vi "charudatta.vi"() -> ()   [LabVIEW 2012]
uses:
  <vilib>/addons/Modulation/Digital/General/MT Generate PSK System Parameters(M).vi
  <instrlib>/niUSRP/niUSRP Write Tx Data (CDB Cluster).vi
  <vilib>/addons/Modulation/Digital/General/MT Generate Bits (Galois, PN Order).vi
  <vilib>/addons/Modulation/niDMT.lvlib
panel:
  out "error out 2":errorcluster caption="error out"
  out "Symbol Rate":dbl
  out "Number of Packets":i32
  in  "Tab Control":T1(tab)
  in  "Message Text":string="Two roads diverged in a yellow wood,\nAnd sorry I could not travel both\nAnd be one traveler, long I stood\nAnd looked down one as far as I could\nTo where it bent in the undergrowth.\n\nThen took the other, as just as fair,\nAnd having perhaps the better claim,\nBecause it was grassy and wanted wear;\nThough as for that the passing there\nHad worn them really about the same.\n\nAnd both that morning equally lay\nIn leaves no step had trodden black.\nOh, I kept the first for another day!\nYet knowing how way leads on to way,\nI doubted if I should ever come back.\n\nI shall be telling this with a sigh\nSomewhere ages and ages hence:\nTwo roads diverged in a wood, and I--\nI took the one less traveled by,\nAnd that has made all the difference.\n"
  in  "Packet Parameters":T2={"Guard Bits "=30, "Sync Bits"=20, "Message Bits"=128}
  in  "Packet Pad \n[samples]":i32=200
  in  "Blank Frame \n[samples]":i32=500
  out "Number of Packets in Message":i32=46
  in  "PN sequence order\nfor Sync Bits":i32=31 caption="PN sequence order (9)"
  in  "Packet Repeat":i32=2
  in  "Select PSK Modulation Format":T3(tab)=enum."QPSK" caption="PSK"
  in  "BPSK System Parameters":T4={"Samples per Symbol"=8, "symbol map"=[], "Differential PSK"=enum."disable", "PSK type"=0} {"PSK type" items=["normal", "shifted", "offset"]; "symbol map" format="%.3f"}
  in  "QPSK System Parameters":T4={"Samples per Symbol"=8, "symbol map"=[], "Differential PSK"=enum."disable", "PSK type"=0} {"PSK type" items=["normal", "shifted", "offset"]; "symbol map" format="%.3f"}
  in  "pi/4 DQPSK System Parameters":T4={"Samples per Symbol"=8, "symbol map"=[], "Differential PSK"=enum."enable", "PSK type"=1} {"PSK type" items=["normal", "shifted", "offset"]; "symbol map" format="%.3f"}
  in  "OQPSK System Parameters":T4={"Samples per Symbol"=8, "symbol map"=[], "Differential PSK"=enum."disable", "PSK type"=2} {"PSK type" items=["normal", "shifted", "offset"]; "symbol map" format="%.3f"}
  in  "8-PSK System Parameters":T4={"Samples per Symbol"=8, "symbol map"=[], "Differential PSK"=enum."disable", "PSK type"=0} {"PSK type" items=["normal", "shifted", "offset"]; "symbol map" format="%.3f"}
  in  "16-PSK System Parameters":T4={"Samples per Symbol"=8, "symbol map"=[], "Differential PSK"=enum."disable", "PSK type"=0} {"PSK type" items=["normal", "shifted", "offset"]; "symbol map" format="%.3f"}
  in  "M":i32=4 min=2 step=2
  in  "Custom System Parameters":T4={"Samples per Symbol"=8, "symbol map"=[], "Differential PSK"=enum."disable", "PSK type"=0} {"PSK type" items=["normal", "shifted", "offset"]; "symbol map" format="%.3f"}
  in  "Pulse Shaping Filter Parameters":T5={"Alpha"=0.5, "Filter Length"=6, "TX Filter"=enum."Root Raised Cos"} caption="Pulse Shaping Filter" {"Alpha" format="%.2f"}
  in  "Tx Parameters":T6={"Tx IQ Sampling\nRate [s/sec]"=500000.0, "Tx Frequency [Hz]"=2500000000.0, "Tx Gain [dB]"=0.0, "Tx Antenna"="TX1"} {"Tx Gain [dB]" format="%#.6p"; "Tx Frequency [Hz]" format="%#.6p"; "Tx IQ Sampling\nRate [s/sec]" format="%#.6p"}
  out "Actual Tx Parameters":T6={"Tx IQ Sampling\nRate [s/sec]"=200000.0, "Tx Frequency [Hz]"=2500000000.0, "Tx Gain [dB]"=0.0, "Tx Antenna"="TX1"} {"Tx Gain [dB]" format="%#.6p"; "Tx Frequency [Hz]" format="%#.6p"; "Tx IQ Sampling\nRate [s/sec]" format="%#.6p"}
  in  "USRP IP address":refnum<k15>="192.168.10.2"
  out "error out":errorcluster
  in  "Queue Length":i32=10
  out "Constellation Graph":T7(graph)
  in  "autoscale":bool
  in  "stop":bool
  # "Guard\nBand"
  # "Sync\nSeq"
  # "Packet\nNumber"
  # "Pad\nData"
  # "Blank\nFrame"
  # "Data"
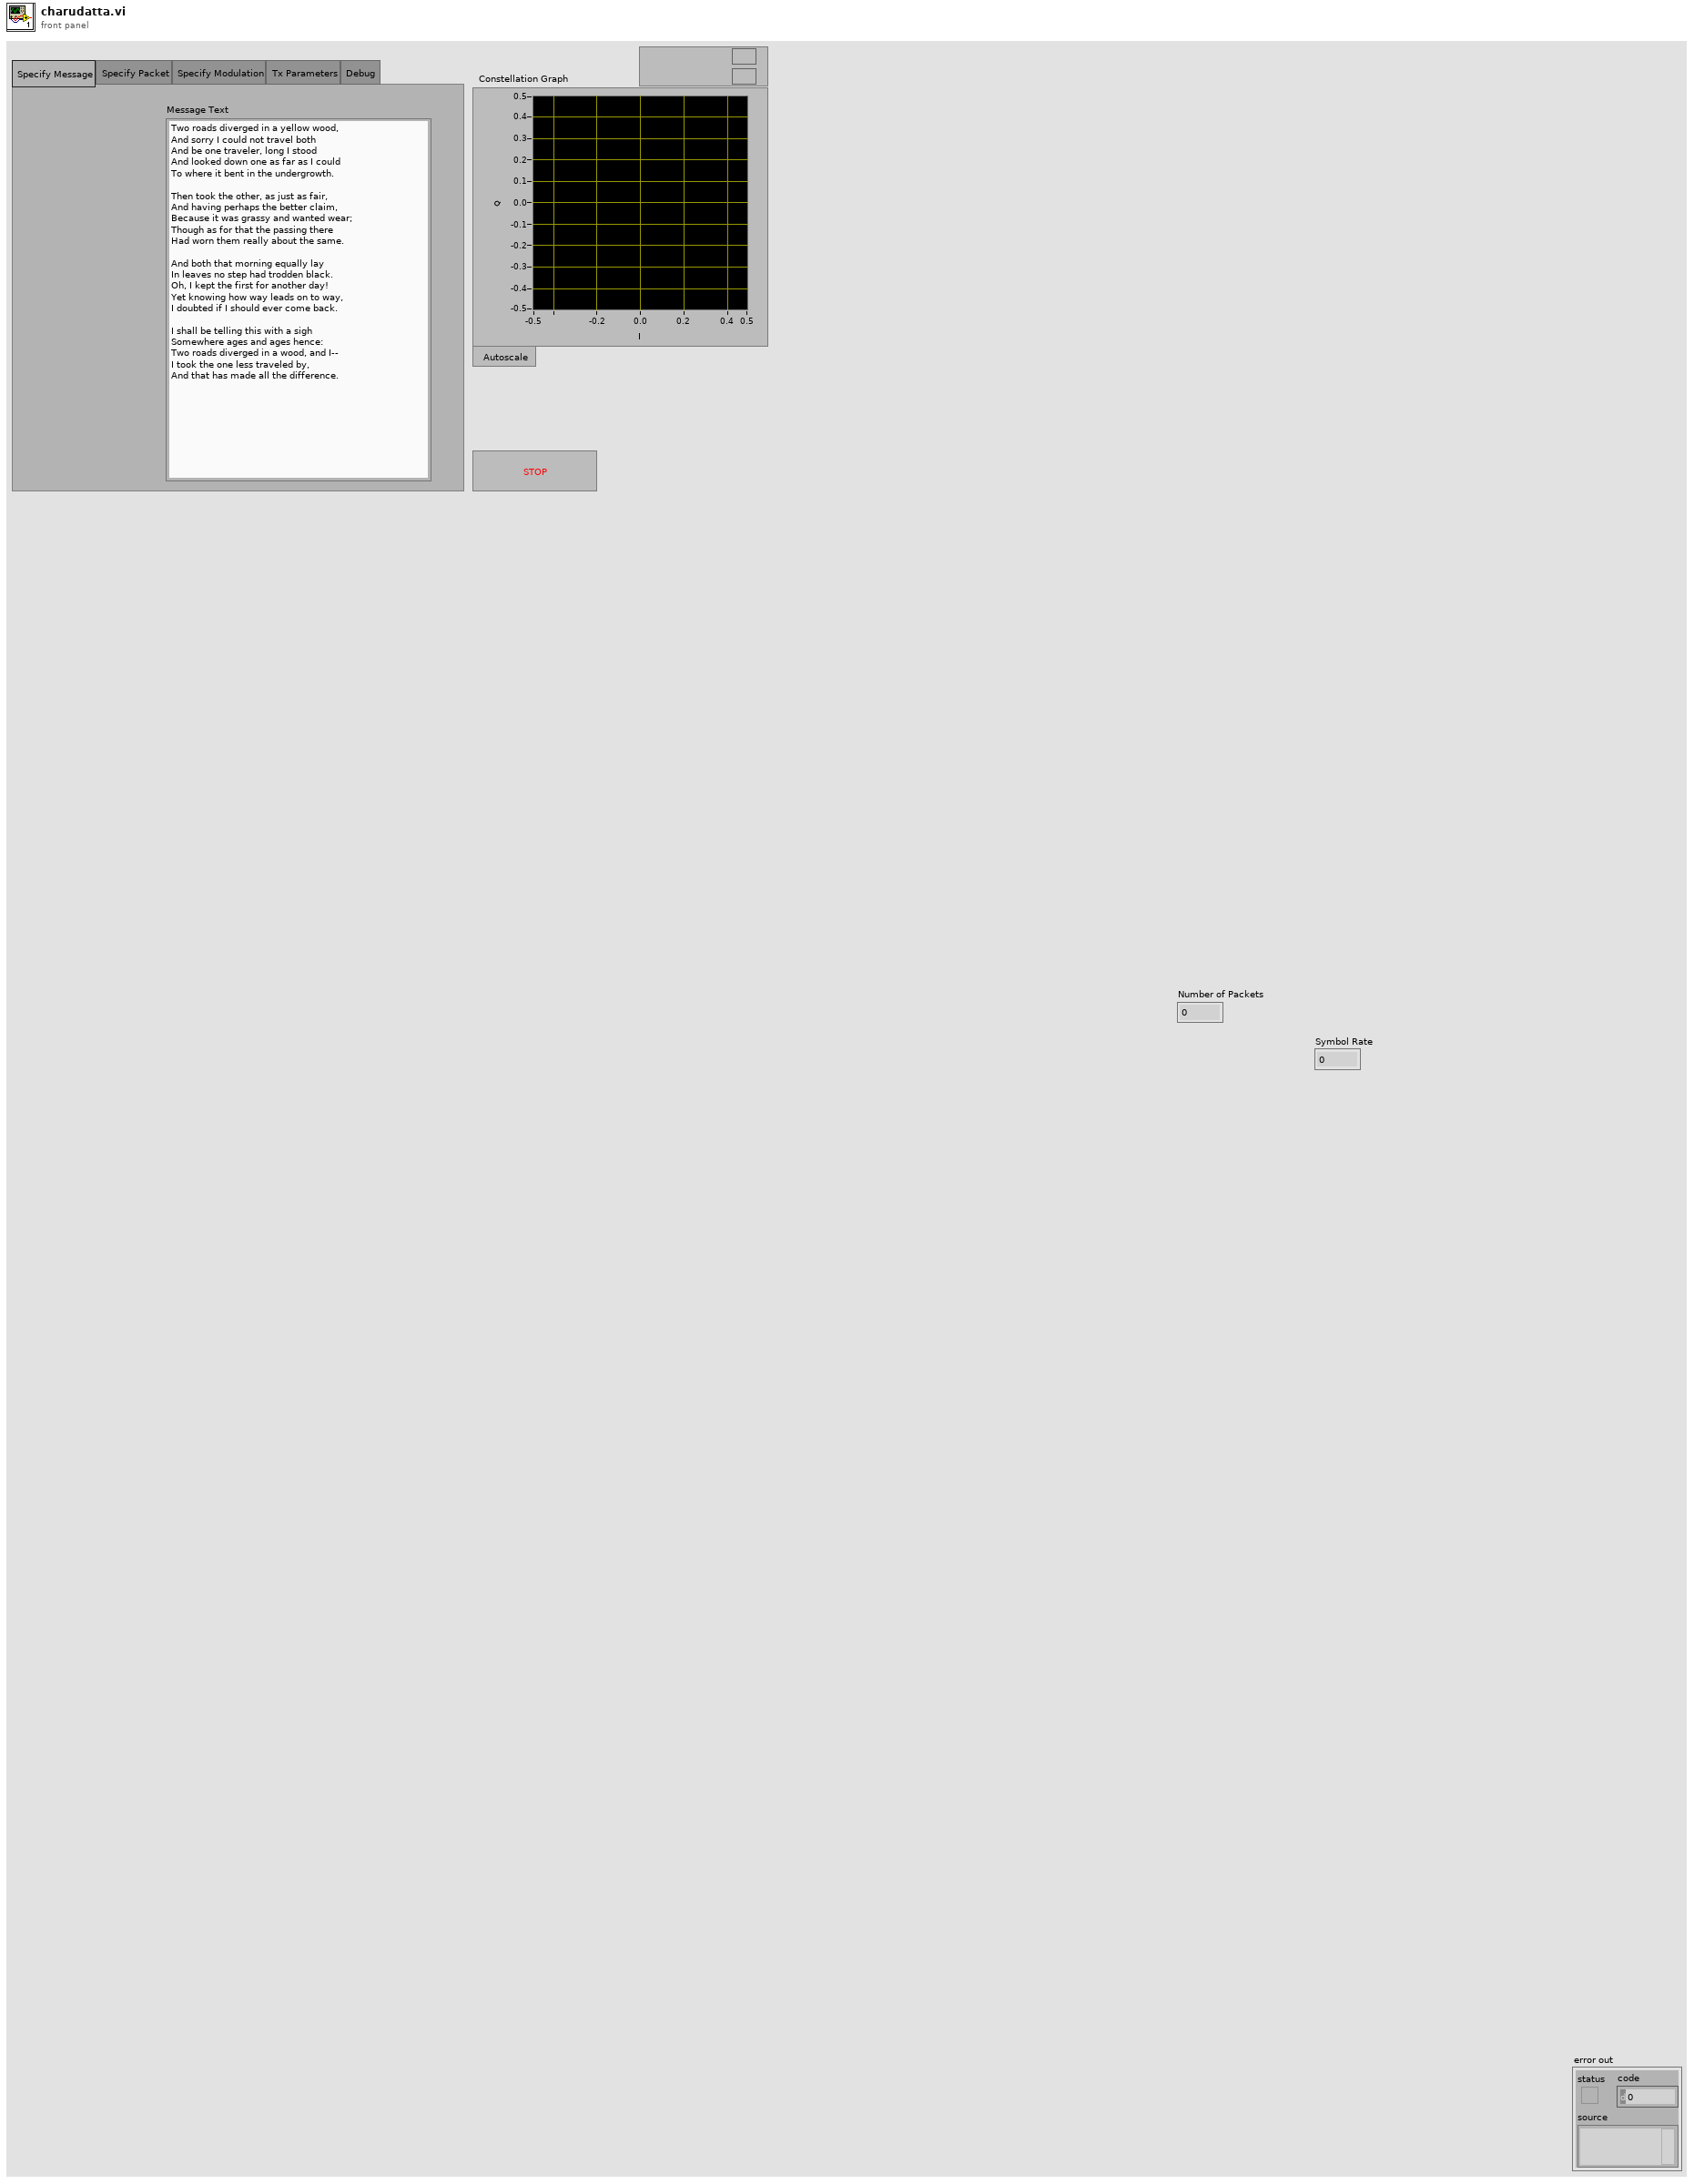
[diagram p1: front panel]
types:
  T1 = enum32{"Specify Message", "Specify Packet", "Specify Modulation", "Tx Parameters", "Debug"}
  T2 = cluster{"Guard Bits ":i32, "Sync Bits":i32, "Message Bits":i32}
  T3 = enum32{"BPSK", "QPSK", "pi/4DQPSK", "OQPSK", "8-PSK", "16-PSK", "Custom"}
  T4 = cluster{"Samples per Symbol":i32, "symbol map":cdb[], "Differential PSK":enum16{"disable", "enable"}, "PSK type":u16}
  T5 = cluster{"Alpha":dbl, "Filter Length":i32, "TX Filter":enum16{"none", "Raised Cosine", "Root Raised Cos", "Gaussian"}}
  T6 = cluster{"Tx IQ Sampling\nRate [s/sec]":dbl, "Tx Frequency [Hz]":dbl, "Tx Gain [dB]":dbl, "Tx Antenna":string}
  T7 = cluster{"Decimated Array":dbl[], "Decimated Array":dbl[]}[]
  T8 = cluster{"samples per symbol (16)":i32, "symbol map":cdb[], "differential PSK":enum16{"disable", "enable"}, "PSK type":u16}
  T9 = cluster{"s? t:f":cluster{"t0":dbl, "dt":dbl, "Y":cdb[]}, i32}
  T10 = cluster{"output complex waveform":cluster{"t0":dbl, "dt":dbl, "Y":cdb[]}, i32}
  T11 = cluster{"constellation":dbl[], "oversampled data":dbl[]}[]
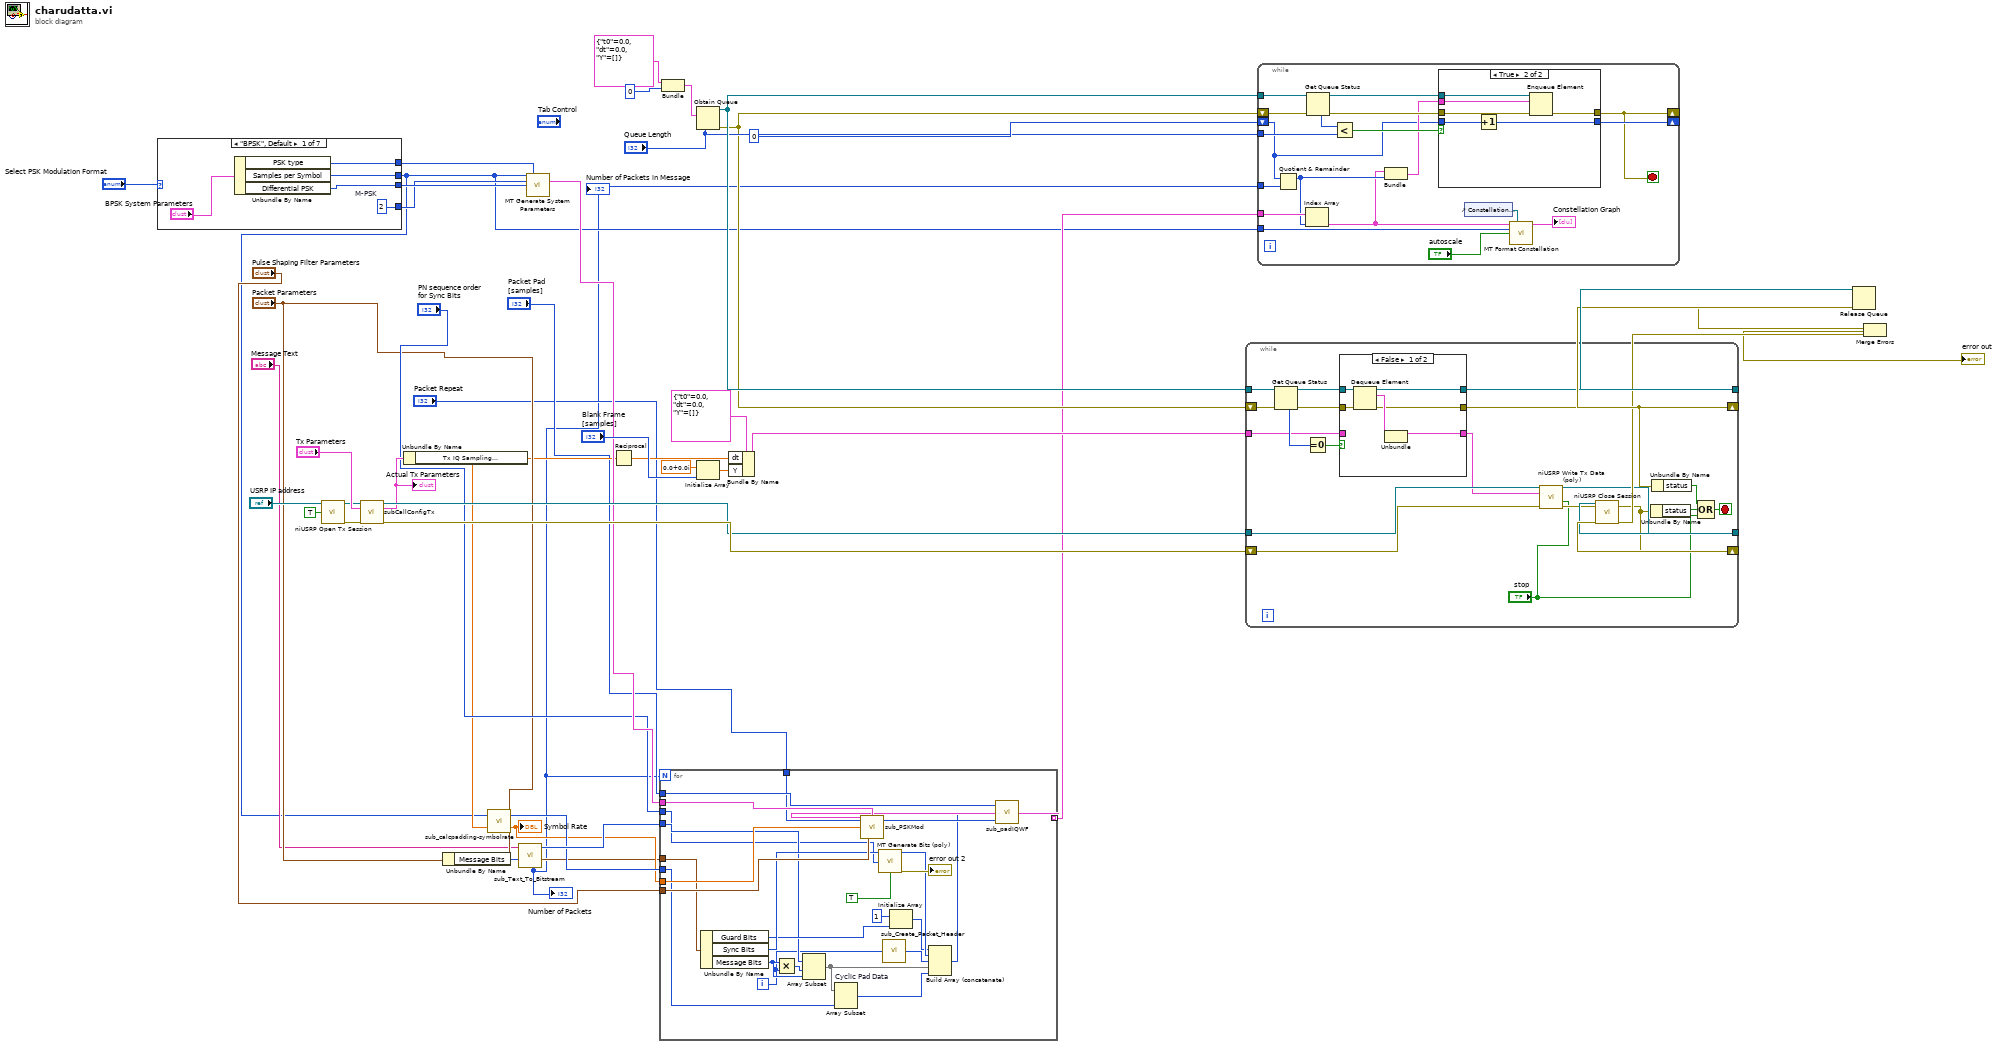
[diagram p0: block diagram]
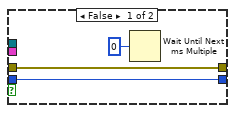
[diagram p2: hidden frame]
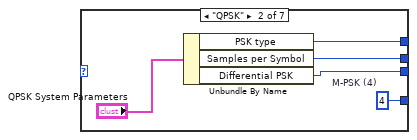
[diagram p3: hidden frame]
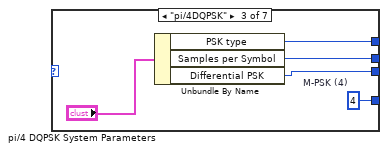
[diagram p4: hidden frame]
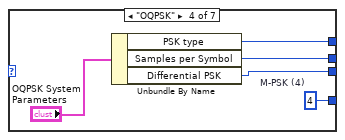
[diagram p5: hidden frame]
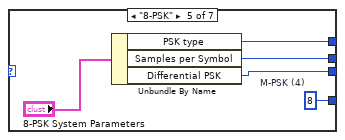
[diagram p6: hidden frame]
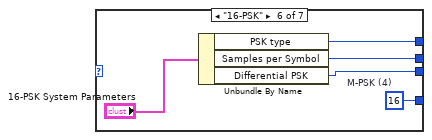
[diagram p7: hidden frame]
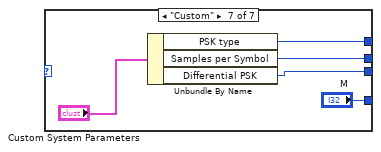
[diagram p8: hidden frame]
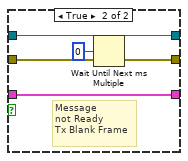
[diagram p9: hidden frame]
diagram:
  n1 = case shown="\"BPSK\", Default" "Select PSK Modulation Format" {
    tunnel: [w49 w53 w61 w66 w71 w77 w80] -> w3
    tunnel: [w50 w55 w60 w65 w70 w76 w81] -> w46
    tunnel: [w52 w57 w62 w67 w69 w75 "M"] -> w29
    tunnel: [w51 w56 w59 w64 w72 w74 w82] -> w20
    frame "BPSK", Default {
      w52 = 2  # M-PSK
      n2 = Unbundle By Name("BPSK System Parameters") -> ("PSK type"=w51:u16, "Samples per Symbol"=w49:i32, "Differential PSK"=w50:enum16{"disable", "enable"})
    }
    frame "QPSK" {
      w57 = 4  # M-PSK (4)
      n3 = Unbundle By Name("QPSK System Parameters") -> ("PSK type"=w56:u16, "Samples per Symbol"=w53:i32, "Differential PSK"=w55:enum16{"disable", "enable"})
    }
    frame "pi/4DQPSK" {
      w62 = 4  # M-PSK (4)
      n4 = Unbundle By Name("pi/4 DQPSK System Parameters") -> ("PSK type"=w59:u16, "Samples per Symbol"=w61:i32, "Differential PSK"=w60:enum16{"disable", "enable"})
    }
    frame "OQPSK" {
      w67 = 4  # M-PSK (4)
      n5 = Unbundle By Name("OQPSK System Parameters") -> ("PSK type"=w64:u16, "Samples per Symbol"=w66:i32, "Differential PSK"=w65:enum16{"disable", "enable"})
    }
    frame "8-PSK" {
      w69 = 8  # M-PSK (4)
      n6 = Unbundle By Name("8-PSK System Parameters") -> ("PSK type"=w72:u16, "Samples per Symbol"=w71:i32, "Differential PSK"=w70:enum16{"disable", "enable"})
    }
    frame "16-PSK" {
      w75 = 16  # M-PSK (4)
      n7 = Unbundle By Name("16-PSK System Parameters") -> ("PSK type"=w74:u16, "Samples per Symbol"=w77:i32, "Differential PSK"=w76:enum16{"disable", "enable"})
    }
    frame "Custom" {
      n8 = Unbundle By Name("Custom System Parameters") -> ("PSK type"=w82:u16, "Samples per Symbol"=w80:i32, "Differential PSK"=w81:enum16{"disable", "enable"})
    }
  }
  n9 = call <instrlib>:"niUSRP Open Tx Session.vi"("device names"="USRP IP address", "reset"=TRUE) -> ("session handle out"=w23:refnum<k15>, "error out"=w22:errorcluster)  [unwired: 12 in]
  n10 = call "subCallConfigTx.vi"("session handle"=w23, "Tx Parameters"="Tx Parameters", "error in"=w22) -> ("session handle out"=w28:refnum<k15>, "Actual Tx Parameters"=w27:T6, "error out"=w33:errorcluster)  [unwired: 10 in]
  "Actual Tx Parameters" <- w27
  n11 = Unbundle By Name(w27) -> ("Tx IQ Sampling\nRate [s/sec]"=w6:dbl)
  n12 = Unbundle By Name("Packet Parameters") -> ("Message Bits"=w14:i32)
  n13 = call "sub_calcpadding-symbolrate.vi"("Tx IQ Sampling\nRate [s/sec]"=w6, "Samples per Symbol"=w3) -> ("Symbol Rate"=w12:dbl, "Padding Bits"=w13:i32)
  "Symbol Rate" <- w12
  n14 = call "sub_Text_To_Bitstream.vi"("Packet\nMessage Length (bits)"=w14, "text"="Message Text") -> ("message bitstream"=w15:i8[], "Number of Packets"=w1:i32)  [unwired: 7 in, 1 out]
  "Number of Packets in Message" <- w1
  "Number of Packets" <- w1
  n15 = call-poly <vilib>:"MT Generate System Parameters.vi"("samples per symbol (16)"=w3, "PSK type"=w20, "M-PSK (4)"=w29, "differential PSK"=w46) -> ("PSK system parameters"=w10:T8)  [unwired: 9 in, 2 out]
  n16 = Reciprocal(x=w6) -> (1/x=w30:dbl)
  n17 = for {
    N: w1 -> [_]
    tunnel: "Packet Parameters" -> [w88]
    tunnel: [w104] -> w11 mode=indexing
    tunnel: w15 -> [w87]
    tunnel: "PN sequence order\nfor Sync Bits" -> [w86]
    tunnel: w13 -> [w84]
    tunnel: w10 -> [w107]
    tunnel: w12 -> [w106]
    tunnel: "Pulse Shaping Filter Parameters" -> [w105]
    tunnel: "Packet Pad \n[samples]" -> [w102]
    tunnel: "Packet Repeat" -> [w101]
    i -> [w85]
    n18 = Unbundle By Name(w88) -> ("Guard Bits"=w92:i32, "Sync Bits"=w98:i32, "Message Bits"=w96:i32)
    n19 = Multiply(x=w96, y=w85) -> (x*y=w89:i32)
    n20 = Array Subset(array=w87, index=w89, length=w96) -> (w94:i8[])
    n21 = Array Subset "Cyclic Pad Data"(array=w94, length=w84) -> (w93:i8[])  [unwired: 1 in]
    n22 = call-poly <vilib>:"MT Generate Bits (poly).vi"("total bits (128)"=w98, "PN sequence order (9)"=w86, "reset? (T)"=TRUE ("Reset? (T)")) -> ("output bit stream"=w95:i8[], "error out"=→"error out 2":errorcluster)  [unwired: 10 in, 1 out]
    n23 = call "sub_Create_Packet_Header.vi"("Packet Number"=w85) -> ("header bits"=w97:i8[])
    n24 = Initialize Array(i8 1 ("Numeric"), w92) -> (w90:i8[])
    n25 = Build Array (concatenate)(w90, w95, w97, w94, w93) -> (w83:i8[])
    n26 = call "sub_PSKMod.vi"("Packet to Transmit"=w83, "PSK system parameters"=w107, "Symbol Rate, Hz"=w106, "filter parameters"=w105) -> ("output complex waveform"=w103:cluster{"t0":dbl, "dt":dbl, "Y":cdb[]})  [unwired: 10 in, 1 out]
    n27 = call "sub_padIQWF.vi"("Repeat"=w101, "input complex waveform"=w103, "Packet Pad \n[samples]"=w102) -> ("output complex waveform"=w104:cluster{"t0":dbl, "dt":dbl, "Y":cdb[]})
  }
  n28 = Bundle("s? t:f"=cluster{"t0":dbl, "dt":dbl, "Y":cdb[]} {"t0"=0.0, "dt"=0.0, "Y"=[]}, 0) -> (w37:T9)  [unwired: 1 in]
  n29 = Obtain Queue(max queue size (-1, unlimited)="Queue Length", element data type=w37) -> (queue out=w43:refnum<queue>, error out=w25:errorcluster)  [unwired: 3 in, 1 out]
  n30 = Initialize Array(cdb 0.0+0.0i ("element"), "Blank Frame \n[samples]") -> (w42:cdb[])
  n31 = Bundle By Name(cluster=cluster{"t0":dbl, "dt":dbl, "Y":cdb[]} {"t0"=0.0, "dt"=0.0, "Y"=[]} ("s? t:f"), "dt"=w30, "Y"=w42) -> (w41:cluster{"t0":dbl, "dt":dbl, "Y":cdb[]})
  n32 = while {
    tunnel: w28 -> [w116]
    shift-right: [w113] -> w32
    shift-left: w33 -> [w117]
    tunnel: w43 -> [w125]
    tunnel: w41 -> [w122]
    tunnel: [w121] -> w40
    tunnel: [w115] -> w31
    shift-right: [w110] -> w39
    shift-left: w25 -> [w118]
    stop <- w112 stop-if-true
    n33 = Get Queue Status(queue=w125, error in (no error)=w118) -> (queue out=w120:refnum<queue>, error out=w119:errorcluster, # elements in queue=w124:i32)  [unwired: 1 in, 5 out]
    n34 = Equal To 0?(x=w124) -> (x = 0?=w123:bool)
    n35 = case shown="False" w123 {
      tunnel: w122 -> [_ w135]
      tunnel: [w127 w135] -> w108
      tunnel: [w131 w133] -> w121
      tunnel: [w126 w134] -> w110
      tunnel: w120 -> [w130 w133]
      tunnel: w119 -> [w129 w134]
      frame False {
        n36 = Dequeue Element(queue=w130, error in (no error)=w129) -> (queue out=w131:refnum<queue>, element=w128:T9, error out=w126:errorcluster)  [unwired: 1 in, 1 out]
        n37 = Unbundle(w128) -> ("s? t:f"=w127:cluster{"t0":dbl, "dt":dbl, "Y":cdb[]})  [unwired: 1 out]
      }
      frame True {
        # "Message\nnot Ready\nTx Blank Frame"
        n38 = Wait Until Next ms Multiple(millisecond multiple=u32 0) -> ()  [unwired: 1 out]
      }
    }
    n39 = call-poly <instrlib>:"niUSRP Write Tx Data (poly).vi"("session handle"=w116, "data"=w108, "end of data?"="stop", "error in (no error)"=w117) -> ("session handle out"=w115:refnum<k15>, "error out"=w113:errorcluster)  [unwired: 10 in]
    n40 = Unbundle By Name(w113) -> ("status"=w114:bool)
    n41 = Unbundle By Name(w110) -> ("status"=w109:bool)
    n42 = Compound Arithmetic op=OR(w109, w114, "stop") -> (w112:bool)
  }
  n43 = while {
    tunnel: w43 -> [w154]
    shift-right: [w147] -> _
    shift-left: 0 -> [w143]
    tunnel: w11 -> [w144]
    tunnel: "Queue Length" -> [w146]
    tunnel: w1 -> [w145]
    shift-right: [w141] -> _
    shift-left: w25 -> [w149]
    tunnel: w3 -> [w138]
    stop <- w141 stop-if-true
    n44 = Quotient & Remainder(x=w143, y=w145) -> (x-y*floor(x/y)=w142:i32)  [unwired: 1 out]
    n45 = Index Array(array=w144, index=w142) -> (element=w136:cluster{"t0":dbl, "dt":dbl, "Y":cdb[]})
    n46 = Get Queue Status(queue=w154, error in (no error)=w149) -> (queue out=w153:refnum<queue>, error out=w150:errorcluster, # elements in queue=w152:i32)  [unwired: 1 in, 5 out]
    n47 = Less?(x=w152, y=w146) -> (x < y?=w151:bool)
    n48 = Bundle("output complex waveform"=w136, w142) -> (w148:T10)  [unwired: 1 in]
    n49 = case shown="True" w151 {
      tunnel: w150 -> [w155 w163]
      tunnel: w153 -> [_ w162]
      tunnel: [w155 w161] -> w141
      tunnel: w148 -> [_ w160]
      tunnel: w143 -> [w157 w159]
      tunnel: [w157 w158] -> w147
      frame False {
        n50 = Wait Until Next ms Multiple(millisecond multiple=u32 0) -> ()  [unwired: 1 out]
      }
      frame True {
        n51 = Increment(x=w159) -> (x+1=w158:i32)
        n52 = Enqueue Element(queue=w162, element=w160, error in (no error)=w163) -> (error out=w161:errorcluster)  [unwired: 1 in, 2 out]
      }
    }
    n53 = control-ref of="Constellation Graph"() -> (w139:refnum<vi>)
    n54 = call <vilib>:"MT Format Constellation.vi"("waveform"=w136, "constellation reference"=w139, "samples per symbol"=w138, "autoscale"="autoscale") -> ("constellation graph"=→"Constellation Graph":T11)  [unwired: 1 in, 10 out]
  }
  n55 = call <instrlib>:"niUSRP Close Session.vi"("session handle"=w31, "error in (no error)"=w32) -> ("error out"=w18:errorcluster)  [unwired: 13 in]
  n56 = Release Queue(queue=w40, error in (no error)=w39) -> (error out=w19:errorcluster)  [unwired: 3 out]
  n57 = Merge Errors(w19, w18) -> (→"error out":errorcluster)
